vi "Convert Error Cluster to Table.vi"(11 "Error Codes":cluster{i32, string}[](array[cluster])) -> (2 "Code":i32[](array[numeric]), 3 "String":string[](array[string]))   [LabVIEW 2019, in "Protection and Counter Addon System Explorer.lvlib"] (continued)
 application instance."}, {1501, "LabVIEW: (Hex 0x5DD) Not a VRML 97 file, or contains unsupported models."}, {1502, "LabVIEW: (Hex 0x5DE) Cannot save a bad VI without its block diagram."}, {1503, "LabVIEW: (Hex 0x5DF) Cannot save a clone of a reentrant VI."}, {1504, "LabVIEW: (Hex 0x5E0) Cannot save a remote panel."}, {1505, "LabVIEW: (Hex 0x5E1) Cannot save a remote-debugging VI."}, {1506, "LabVIEW: (Hex 0x5E2) Cannot save a VI that is being edited in another context."}, {1507, "LabVIEW: (Hex 0x5E3) Cannot change the name or path of a VI in its current state."}, {1508, "LabVIEW: (Hex 0x5E4) Cannot change the name or path of a VI that is part of a library in its current state."}, {1509, "LabVIEW: (Hex 0x5E5) The response from the NI Service Locator is not a valid HTTP response."}, {1510, "LabVIEW: (Hex 0x5E6) The requested service was not found as a registered service with the NI Service Locator."}, {1511, "LabVIEW: (Hex 0x5E7) The requested service is a registered service with the NI Service Locator but it did not contain a port mapping."}, {1512, "LabVIEW: (Hex 0x5E8) trying to set indexes of bundle/unbundle with an array that is too long"}, {1513, "LabVIEW: (Hex 0x5E9) trying to set indexes of bundle/unbundle with an array that is too short"}, {1514, "LabVIEW: (Hex 0x5EA) trying to set index of bundle/unbundle to an element not in the cluster"}, {1515, "LabVIEW: (Hex 0x5EB) Cannot access this property because the conditional terminal has not been created."}, {1516, "LabVIEW: (Hex 0x5EC) The method in the DLL overwrote the space allocated for one of its parameters. This may have corrupted memory."}, {1517, "LabVIEW: (Hex 0x5ED) An error occurred in the Call Library Node processing. This error was most likely a configuration mismatch between the calling conventions of the Call Library Node and the function being called in the DLL."}, {1518, "LabVIEW: (Hex 0x5EE) Cannot find default printer. Make sure you have installed and selected a default printer."}, {1519, "LabVIEW: (Hex 0x5EF) Unable to print. Make sure you have installed a printer."}, {1520, "LabVIEW: (Hex 0x5F0) Font not found. LabVIEW cannot find the font at the specified path, or the font is not a True Type (.ttf) font."}, {1521, "LabVIEW: (Hex 0x5F1) Cannot read the value of a control that contains placeholder data."}, {1522, "LabVIEW: (Hex 0x5F2) You can write the Data Binding:Path property only if the control is already bound to a PSP URL."}, {1523, "LabVIEW: (Hex 0x5F3) Passed an invalid number of strings to the Strings [ ] property. You must pass either 1 string or 6 strings."}, {1524, "LabVIEW: (Hex 0x5F4) The target version for save is not formatted correctly."}, {1525, "LabVIEW: (Hex 0x5F5) You cannot read the value of a control when the class that defines the data is not available. You must load a missing LabVIEW class file to make this data readable."}, {1526, "LabVIEW: (Hex 0x5F6) This property does not apply when the plot legend of a graph or chart is in tree view."}, {1527, "LabVIEW: (Hex 0x5F7) Attempted to read flattened data of a LabVIEW class that is not currently loaded into LabVIEW."}, {1528, "LabVIEW: (Hex 0x5F8) A scene object with the specified name was not found."}, {1529, "LabVIEW: (Hex 0x5F9) There are too many nested VI calls. This typically results from recursion without a proper termination condition to stop the recursion."}, {1530, "LabVIEW: (Hex 0x5FA) The running VI attempted to make a subVI call into a top-level VI. LabVIEW does not allow calls into top-level VIs."}, {1531, "LabVIEW: (Hex 0x5FB) The LabVIEW class data cannot be unflattened because the class is broken. You must fix problems with the class before LabVIEW can unflatten data of this class."}, {1532, "LabVIEW: (Hex 0x5FC) The target application instance is currently being destroyed. You cannot get a new reference to the application instance or load a VI in the application instance."}, {1533, "LabVIEW: (Hex 0x5FD) A shared variable node cannot be created from the specified terminal."}, {1534, "LabVIEW: (Hex 0x5FE) The semaphore you specified does not exist. LabVIEW cannot return a reference to the semaphore."}, {1535, "LabVIEW: (Hex 0x5FF) The semaphore reference you specified is invalid."}, {1536, "LabVIEW: (Hex 0x600) To save a password-protected VI for a previous LabVIEW version, you must enter the password."}, {1537, "LabVIEW: (Hex 0x601) Member VI is not dynamic dispatch."}, {1538, "LabVIEW: (Hex 0x602) To perform this operation you must have the LabVIEW Statechart Module installed."}, {1539, "LabVIEW: (Hex 0x603) Valid stipple factors are 1 - 256"}, {1540, "LabVIEW: (Hex 0x604) Cannot pass a degenerate vector for the normal of an object."}, {1541, "LabVIEW: (Hex 0x605) This property or method is not valid because the object is not billboarded."}, {1542, "LabVIEW: (Hex 0x606) You must set the drawable of the object before you configure billboard parameters."}, {1543, "LabVIEW: (Hex 0x607) Cannot pass an empty position list for billboarding."}, {1544, "LabVIEW: (Hex 0x608) LabVIEW attempted a read, write, or seek on a file opened in unbuffered mode, and the data size is not a multiple of the disk sector size."}, {1545, "LabVIEW: (Hex 0x609) LabVIEW attempted to read or write data to a file opened in unbuffered mode, and the data is not aligned properly."}, {1546, "LabVIEW: (Hex 0x60A) The VI must be in a project to use this property."}, {1547, "LabVIEW: (Hex 0x60B) There was an error generating the type library."}, {1548, "LabVIEW: (Hex 0x60C) Queue refnum cannot be obtained with a size of zero. Size input must be a positive number or -1 for unlimited size."}, {1549, "LabVIEW: (Hex 0x60D) An unexpected error occurred during statechart code generation."}, {1550, "LabVIEW: (Hex 0x60E) The license for the I/O server type is invalid."}, {1553, "LabVIEW: (Hex 0x611) The LabVIEW Run-Time Engine cannot load the polymorphic VI. This error occurs in stand-alone applications when the VI is polymorphic."}, {1554, "LabVIEW: (Hex 0x612) The current LabVIEW target cannot load control VIs."}, {1555, "LabVIEW: (Hex 0x613) Property or invoke node is corrupt."}, {1556, "LabVIEW: (Hex 0x614) The reference is invalid. This error might occur because the reference has been deleted."}, {1557, "LabVIEW: (Hex 0x615) LabVIEW tried to access duplicate references at the same time."}, {1558, "LabVIEW: (Hex 0x616) There is a type mismatch between the wire type and the internal data type of the reference. This problem might occur due to a type cast error."}, {1559, "LabVIEW: (Hex 0x617) You cannot use Open VI Reference to create a reference to a VI that the creating VI accesses through community scope."}, {1560, "LabVIEW: (Hex 0x618) A library cannot list itself as a friend."}, {1561, "LabVIEW: (Hex 0x619) A library cannot list an item from a foreign application instance as a friend."}, {1562, "LabVIEW: (Hex 0x61A) The specified project or library is locked."}, {1563, "LabVIEW: (Hex 0x61B) LabVIEW did not generate documentation files for the statechart. Ensure all configuration windows are closed."}, {1564, "LabVIEW: (Hex 0x61C) Project file cannot be saved at this time. The project has a locked untitled dependency. The lock prevents giving the untitled item a name so it cannot be saved."}, {1565, "LabVIEW: (Hex 0x61D) LabVIEW cannot save the library file at this time. The library has a locked untitled dependency. The lock prevents giving the untitled item a name, which is required to save the library file."}, {1566, "LabVIEW: (Hex 0x61E) LabVIEW cannot save the untitled library file at this time. The library is locked. The lock prevents giving the untitled library a name, which is required to save the library."}, {1567, "LabVIEW: (Hex 0x61F) The control is not located in the same VI as the control reference."}, {1568, "LabVIEW: (Hex 0x620) This method requires Excel to be installed."}, {1569, "LabVIEW: (Hex 0x621) This method requires DIAdem 8.1 or later to be installed."}, {1570, "LabVIEW: (Hex 0x622) This method requires the array to be of numeric or string type."}, {1571, "LabVIEW: (Hex 0x623) You cannot open a packed library saved in a version earlier than the current version of LabVIEW."}, {1572, "LabVIEW: (Hex 0x624) The long name of the property is not unique."}, {1573, "LabVIEW: (Hex 0x625) You cannot load a packed library built for a target or operating system different than the current target or operating system."}, {1574, "LabVIEW: (Hex 0x626) Cannot open a file with separated compiled code in the LabVIEW Run-Time Engine."}, {1575, "LabVIEW: (Hex 0x627) The function name for the %s node cannot be found in the library. To correct this error, right-click the Call Library Function Node and select Configure from the shortcut menu. Then choose the correct function name."}, {1576, "LabVIEW: (Hex 0x628) A Start Asynchronous Call node received a reference input that was not configured to allow asynchronous calls. To fix this error, include either the 0x80 option flag or the 0x100 option flag when you open the reference with the Open VI Reference function."}, {1577, "LabVIEW: (Hex 0x629) A Wait On Asynchronous Call node received a reference input that was not configured to wait on an asynchronous call. To fix this error, include the 0x100 option flag when you open the VI reference with the Open VI Reference function."}, {1578, "LabVIEW: (Hex 0x62A) Asynchronous calls are not allowed on remote VI references."}, {1579, "LabVIEW: (Hex 0x62B) Specified paths do not share a common directory."}, {1580, "LabVIEW: (Hex 0x62C) Cannot find the compiled code in the compiled object cache."}, {1581, "LabVIEW: (Hex 0x62D) Cannot use this property on either .NET or ActiveX Container."}, {1582, "LabVIEW: (Hex 0x62E) Cannot call (Target)SaveInstrument on an Inline VI with Save Level greater than 0."}, {1583, "LabVIEW: (Hex 0x62F) LabVIEW Real-Time target is already connected to a host VI. You cannot initiate a remote panel connection to a Real-Time target while also using a host VI to connect to the target. Choose only one method to connect to the target."}, {1584, "LabVIEW: (Hex 0x630) The data in the reference cannot be resized. There is a size mismatch between the data in the reference and the data wired to the Data Value Reference Write Element border node."}, {1585, "LabVIEW: (Hex 0x631) The class library is loaded, but its datatype is not ready to be instantiated."}, {1586, "LabVIEW: (Hex 0x632) Compiled code is out of date."}, {1587, "LabVIEW: (Hex 0x633) VI is not marked to separate compiled code from source file."}, {1588, "LabVIEW: (Hex 0x634) Compiled object cache is corrupt."}, {1589, "LabVIEW: (Hex 0x635) The loaded .NET assembly was not found in its original directory."}, {1590, "LabVIEW: (Hex 0x636) The qualified name of one of the dependencies of the specified file is not what LabVIEW expected. This mismatch implies that the dependency report is unreliable, so the ReadLinkInfo operation was aborted."}, {1591, "LabVIEW: (Hex 0x637) The 0x40 option flag is not valid for either the target VI or the other option flags of the Open VI Reference function."}, {1592, "LabVIEW: (Hex 0x638) The asynchronous option flags require a strictly typed VI reference for the type specifier input of the Open VI Reference function."}, {1593, "LabVIEW: (Hex 0x639) Only one asynchronous call option can be passed into an Open VI Reference at a time."}, {1594, "LabVIEW: (Hex 0x63A) This VI type does not support inlining."}, {1595, "LabVIEW: (Hex 0x63B) The RT target does not have enough memory to load the startup application."}, {1596, "LabVIEW: (Hex 0x63C) Cannot use SSL on this operating system because SSL is either not configured, not installed, or not supported."}, {1597, "LabVIEW: (Hex 0x63D) The Paste Data operation attempted to paste data into a destination that would have had a dimmed 'paste' option in the shortcut menu."}, {1598, "LabVIEW: (Hex 0x63E) The requested path does not match a LabVIEW class in memory."}, {1599, "LabVIEW: (Hex 0x63F) An empty string is not a valid method name."}, {1600, "LabVIEW: (Hex 0x640) The specified method was not found on the specified LabVIEW class."}, {1601, "LabVIEW: (Hex 0x641) Although the requested class (or one of its ancestors) does have a member VI of the requested name, that VI is not actually a method. Either it has no input terminal of the class type or it is a non-runnable kind of VI, like a global VI, control VI, or poly VI."}, {1602, "LabVIEW: (Hex 0x642) The value supplied for the enum input is not supported on this method or property."}, {1603, "LabVIEW: (Hex 0x643) The Open VI Reference function does not support using an asynchronous call by reference option with the <b>Prepare for reentrant run</b> option."}, {1604, "LabVIEW: (Hex 0x644) The Open VI Reference function does not support using the option 0x08 (<b>Prepare for reentrant run</b>) with the asynchronous call by reference options 0x80 (<b>Prepare to call and forget</b>) or 0x100 (<b>Prepare to call and collect</b>)."}, {1605, "LabVIEW: (Hex 0x645) A process attempted to send a message with an invalid priority."}, {1606, "LabVIEW: (Hex 0x646) While attempting to launch, an actor's <b>Pre Launch Init</b> method failed."}, {1607, "LabVIEW: (Hex 0x647) Invalid message enqueuer wired to Actor.lvclass:Launch Actor.vi."}, {1608, "LabVIEW: (Hex 0x648) This actor stopped because it received an emergency stop message."}, {1609, "LabVIEW: (Hex 0x649) This class cannot load into this application instance."}, {1610, "LabVIEW: (Hex 0x64A) The To-Caller and To-Self queues for this actor already are initialized."}, {1611, "LabVIEW: (Hex 0x64B) An internal error occurred because a front panel item has no execute data. Recompiling the VI may fix this issue."}, {1612, "LabVIEW: (Hex 0x64C) You attempted to invoke a dynamic dispatch VI statically. The object you supplied for the dynamic dispatch terminal has an override VI for the chosen method that is not the same as the VI you specified. LabVIEW does not allow callers to directly invoke ancestor versions of the object's method."}, {1613, "LabVIEW: (Hex 0x64D) Calls to remote application instances are not supported for dynamic dispatch VIs."}, {1614, "LabVIEW: (Hex 0x64E) LabVIEW could not create a class with the name you specified. A class with that name already exists."}, {1615, "LabVIEW: (Hex 0x64F) LabVIEW cannot build a path to an .rtm file from the VI being saved."}, {1616, "LabVIEW: (Hex 0x650) The path to save the report is not valid. A valid path cannot contain any of the following characters: <b>(Windows)</b> < > / | : \" * ? or <b>(OS X/Linux)</b> < > \\ | : \" * ?."}, {1617, "LabVIEW: (Hex 0x651) LabVIEW is unable to generate a VI comparison report. Make sure you have write permission to the path you specified and generate the report again."}, {1619, "LabVIEW: (Hex 0x653) LabVIEW is unable to find the Microsoft Word components. Make sure you installed Microsoft Word correctly."}, {1620, "LabVIEW: (Hex 0x654) LabVIEW is unable to create the Microsoft Word report. Try generating the report again. If the problem persists, contact National Instruments technical support."}, {1621, "LabVIEW: (Hex 0x655) LabVIEW is unable to create the Microsoft Word report. Try generating the report again. If the problem persists, contact National Instruments technical support."}, {1622, "LabVIEW: (Hex 0x656) LabVIEW is unable to create the Microsoft Word report. Make sure you installed Microsoft Word correctly and create the report again."}, {1623, "LabVIEW: (Hex 0x657) LabVIEW is unable to find the Microsoft Word components. Make sure you installed Microsoft Word correctly."}, {1624, "LabVIEW: (Hex 0x658) You can only generate web page or plain text reports on OS X and Linux."}, {1625, "LabVIEW: (Hex 0x659) LabVIEW is unable to create a report in the format that you specify. Make sure the report file extension that you entered is one of the following extensions: .xml, .txt, and <b>(Windows)</b> .doc."}, {1626, "LabVIEW: (Hex 0x65A) Unable to disconnect this control from the type definition. The type definition may belong to a library that requires activation."}, {1627, "LabVIEW: (Hex 0x65B) The control index at position %d is invalid."}, {1628, "LabVIEW: (Hex 0x65C) LabVIEW cannot convert the input data type at position %d to the control data type."}, {1629, "LabVIEW: (Hex 0x65D) The control must have a terminal on the block diagram.."}, {1630, "LabVIEW: (Hex 0x65E) If you wire a variant or a LabVIEW class library file (.lvclass) to this function, you must call the function on a VI in the same application instance."}, {1631, "LabVIEW: (Hex 0x65F) Library not found. This VI does not belong to a library, or the library was removed from disk."}, {1632, "LabVIEW: (Hex 0x660) You cannot insert a custom control directly into a subpanel. Use a VI with the custom control on its front panel instead."}, {1633, "LabVIEW: (Hex 0x661) The LabVIEW Real-Time process encountered an unexpected error and restarted automatically."}, {1634, "LabVIEW: (Hex 0x662) The debug feature of the Actor Framework to automatically open the front panel of the Actor Core VI is not supported in the run-time engine. You must add code to your actor's Actor Core VI to open and close its own panel."}, {1635, "LabVIEW: (Hex 0x663) LabVIEW failed to invoke the Xcode toolchain. Make sure you installed Xcode properly and have signed the Xcode license agreement."}, {1636, "LabVIEW: (Hex 0x664) The SSE settings of the target or operating system does not match the settings of a VI in the application you are trying to build. That VI cannot recompile because it does not have a block diagram."}, {1637, "LabVIEW: (Hex 0x665) This operation cannot be performed on reentrant clone VIs."}, {1638, "LabVIEW: (Hex 0x666) Muliple errors occurred upstream. No details are available (error information may have been deleted somewhere along the way)."}, {1639, "LabVIEW: (Hex 0x667) The test harness actor executed for longer time than the timeout specified. It was stopped with an Emergency Stop message."}, {1640, "LabVIEW: (Hex 0x668) Channels are incompatible with asynchronous call by reference options 0x80 (<b>Prepare for call-and-forget</b>) and 0x100 (<b>Prepare for call-and-collect</b>)."}, {1641, "LabVIEW: (Hex 0x669) LabVIEW was asked to create a channel for an undefined type, such as an array with no subtype or a missing typedef."}, {1642, "LabVIEW: (Hex 0x66A) LabVIEW attempted to recreate a missing channel endpoint, but the channel template does not have an endpoint of this name. The channel template may have been edited to remove support for this endpoint."}, {1643, "LabVIEW: (Hex 0x66B) The requested channel template does not support the requested transmission type. Some channels only support types that have specific abilities. For example, the Accumulator requires a numeric type so the values may be added up. This error also may occur if the channel template itself is flawed and producing broken code for all requested types."}, {1644, "LabVIEW: (Hex 0x66C) The new name used to rename is the same as the name of data already existing in group."}, {1645, "LabVIEW: (Hex 0x66D) The input data does not exist."}, {1646, "LabVIEW: (Hex 0x66E) The source element type cannot be converted to the destination element type."}, {1647, "LabVIEW: (Hex 0x66F) The plot type cannot be mapped to TDMS channels."}, {1648, "LabVIEW: (Hex 0x670) This VI halted execution when attempting to read from or write to a channel wire. The channel includes a branch not connected to a channel endpoint. All branches of a channel wire must be connected to a channel endpoint, either in this block diagram or in the block diagram of a calling VI if the channel is passed out through the connector pane."}, {1649, "LabVIEW: (Hex 0x671) The data carried by a channel wire must be of a public data type. You are trying to create a channel of a typedef or class that uses an access scope other than public or is inside a non-public library."}, {1650, "LabVIEW: (Hex 0x672) LabVIEW.exe not found. Make sure the configured LabVIEW is present under Program Files/Program Files(x86)->National Instruments-><Specific LabVIEW version>->LabVIEW.exe."}, {1651, "LabVIEW: (Hex 0x673) Other instances of LabVIEW might be open and holding the network resources. Close all instances of the configured LabVIEW and try again."}, {1652, "LabVIEW: (Hex 0x674) The network connection was closed. This can happen if the LabVIEW process is killed manually or the firewall restricted/closed the network connection."}, {1653, "LabVIEW: (Hex 0x675) The configured VI is not found. Reconfigure the VI Interop node to point to proper location."}, {1654, "LabVIEW: (Hex 0x676) Failed to launch LabVIEW. Make sure you can run configured LabVIEW. Contact National Instruments for technical support."}, {1655, "LabVIEW: (Hex 0x677) VI Interop node did not execute as expected. Contact National Instruments for technical support."}, {1656, "LabVIEW: (Hex 0x678) Connector pane of the configured VI has changed since VI Interop node was configured. Try reloading the caller VI."}, {1657, "LabVIEW: (Hex 0x679) The component reference is invalid."}, {1658, "LabVIEW: (Hex 0x67A) A Type Specialization structure cannot be assigned a default frame. The last frame will be used if all earlier frames are broken."}, {1659, "LabVIEW: (Hex 0x67B) A Type Specialization structure cannot have conditions assigned to its frames."}, {1660, "LabVIEW: (Hex 0x67C) Cannot set the Active Frame property on a Type Specialization structure. The Active Frame is computed automatically by choosing the first unbroken frame, defaulting to the last frame if all are broken."}, {1661, "LabVIEW: (Hex 0x67D) The NI Python Interface DLL niPythonInterface.dll could not be loaded."}, {1662, "LabVIEW: (Hex 0x67E) The NI Python Host EXE niPythonHost.exe could not be found."}, {1663, "LabVIEW: (Hex 0x67F) Unable to load the Python interpreter of the specified version. Ensure that you install the supported versions of Python, and the bitness of Python matches the bitness of LabVIEW that opens the Python session."}, {1664, "LabVIEW: (Hex 0x680) The specified Python version is not supported."}, {1665, "LabVIEW: (Hex 0x681) The specified Python path is not valid."}, {1666, "LabVIEW: (Hex 0x682) The Python session refnum input is not valid."}, {1667, "LabVIEW: (Hex 0x683) The specified Python module could not be imported."}, {1668, "LabVIEW: (Hex 0x684) The specified Python function could not be found in the specified module."}, {1669, "LabVIEW: (Hex 0x685) The operation to convert from LabVIEW objects to Python objects failed."}, {1670, "LabVIEW: (Hex 0x686) The operation to convert from Python objects to LabVIEW objects failed."}, {1671, "LabVIEW: (Hex 0x687) There was an error in executing the specified function."}, {1672, "LabVIEW: (Hex 0x688) There was an unknown Python error in the operation."}, {1673, "LabVIEW: (Hex 0x689) The VI is not loaded in memory. To load the VI into memory on the server, manually open the VI or use Open VI Reference."}, {1674, "LabVIEW: (Hex 0x68A) The peer closed the network connection. To configure access on the server side for the machine, navigate to Tools>>Options>>VI Server."}, {1675, "LabVIEW: (Hex 0x68B) The input string contains one or more invalid UTF-8 string sequences."}, {1676, "LabVIEW: (Hex 0x68C) A Start Asynchronous Call node received a reference input that is not configured to allow asynchronous calls. When you open the reference with the Open VI Reference node, select \"Prepare for asynchronous call without wait\" or \"Prepare for asynchronous call with wait\"."}, {1677, "LabVIEW: (Hex 0x68D) A Wait On Asynchronous Call node received a reference input that is not configured to wait on an asynchronous call. When you open the VI reference with the Open VI Reference node, select \"Prepare for asynchronous call with wait\"."}, {1678, "LabVIEW: (Hex 0x68E) EnableSimultaneousCalls is not valid for either the target VI or the other call options of the Open VI Reference."}, {1679, "LabVIEW: (Hex 0x68F) Component of the specified name is not in memory."}, {1680, "LabVIEW: (Hex 0x690) The text read from the file contains one or more invalid UTF-8 string sequences."}, {1681, "LabVIEW: (Hex 0x691) Operation attempted to update element, key, or value data in set or map controls. No data operation is allowed for controls inside a set or map."}, {1682, "LabVIEW: (Hex 0x692) The string contains an unexpected null character."}, {1690, "LabVIEW: (Hex 0x69A) Cannot insert the panel of a VI in a panel container if the VI is not running."}, {1691, "LabVIEW: (Hex 0x69B) Cannot insert the panel of a VI in a panel container if the panel is already displayed in a window or another panel container."}, {1692, "LabVIEW: (Hex 0x69C) Inserting this panel results in a cyclic dependency between panel containers."}, {1800, "LabVIEW: (Hex 0x708) Start time input is not an integer multiple of dt. Value was coerced to nearest integer multiple of dt."}, {1801, "LabVIEW: (Hex 0x709) Duration input is not an integer multiple of dt. Value was coerced to nearest integer multiple of dt."}, {1802, "LabVIEW: (Hex 0x70A) Waveforms have different dt values."}, {1803, "LabVIEW: (Hex 0x70B) Waveform x-axis value requested is out of range."}, {1804, "LabVIEW: (Hex 0x70C) Start index, value, or tolerance is NaN."}, {1805, "LabVIEW: (Hex 0x70D) Start index is out of range."}, {1806, "LabVIEW: (Hex 0x70E) Signal value input is outside the range of the digital data."}, {1807, "LabVIEW: (Hex 0x70F) Appending data with mismatched numbers of digital samples or signals."}, {1808, "LabVIEW: (Hex 0x710) Values other than 0, 1, L, H are present in the digital data."}, {1809, "LabVIEW: (Hex 0x711) Highest resolution supported for conversion is 52."}, {1814, "LabVIEW: (Hex 0x716) Values other than 0, 1, L, and H are present in the digital data and were coerced to 0."}, {2300, "LabVIEW: (Hex 0x8FC) The model code of the target is different than the model code of the image."}, {2301, "LabVIEW: (Hex 0x8FD) The image is invalid."}, {2302, "LabVIEW: (Hex 0x8FE) The operation cannot be completed because the target is locked."}, {2303, "LabVIEW: (Hex 0x8FF) The version of the image is not compatible with the version of the system replication VIs."}, {2304, "LabVIEW: (Hex 0x900) The command is not supported on the target."}, {2305, "LabVIEW: (Hex 0x901) The target did not restart because it is already in Install Mode."}, {2306, "LabVIEW: (Hex 0x902) The format command failed. If your target has a Safe Mode dip switch, make sure that it is enabled and try the format command again."}, {2307, "LabVIEW: (Hex 0x903) Failed to remove files or folders."}, {2308, "LabVIEW: (Hex 0x904) Found no configured network adapters."}, {2535, "LabVIEW: (Hex 0x9E7) Data from TDMS files is read using the byte order of the host system. Byte order settings that differ from the host order are ignored."}, {2552, "LabVIEW: (Hex 0x9F8) This property does not contain data."}, {2901, "LabVIEW: (Hex 0xB55) The source control operation was cancelled before completion."}, {2902, "LabVIEW: (Hex 0xB56) A change occurred to the specified file while the operation was running. Reload the file."}, {4800, "LabVIEW: (Hex 0x12C0) Selected Device is Invalid"}, {4801, "LabVIEW: (Hex 0x12C1) Invalid sound task refnum."}, {4802, "LabVIEW: (Hex 0x12C2) The sound device is busy."}, {4803, "LabVIEW: (Hex 0x12C3) The sound driver or card cannot accommodate the specified configuration.  Check that the parameters entered are within the supported range for the hardware and drivers."}, {4804, "LabVIEW: (Hex 0x12C4) Cannot write in file playback."}, {4805, "LabVIEW: (Hex 0x12C5) Could not find the sound file."}, {4806, "LabVIEW: (Hex 0x12C6) DirectX 8.0 or higher is required to run."}, {4810, "LabVIEW: (Hex 0x12CA) Cannot recognize sound format."}, {4811, "LabVIEW: (Hex 0x12CB) Cannot support sound format."}, {4820, "LabVIEW: (Hex 0x12D4) A buffer underflow has occurred."}, {4821, "LabVIEW: (Hex 0x12D5) Overwrite error."}, {4822, "LabVIEW: (Hex 0x12D6) A timeout occurred before the operation finished."}, {4823, "LabVIEW: (Hex 0x12D7) You cannot perform this operation without an active task.  Ensure that a task is active and try again. An input task might stop running if the input buffer overflows. Overflow occurs when the data is not read fast enough."}, {14001, "LabVIEW: (Hex 0x36B1) Invalid refnum."}, {14002, "LabVIEW: (Hex 0x36B2) Invalid string."}, {14003, "LabVIEW: (Hex 0x36B3) A request for a synchronous advise transaction has timed out."}, {14004, "LabVIEW: (Hex 0x36B4) The response to the transaction caused the DDE_FBUSY bit to be set."}, {14005, "LabVIEW: (Hex 0x36B5) A request for a synchronous data transaction has timed out."}, {14006, "LabVIEW: (Hex 0x36B6) The DDEML function was called without first calling the DdeInitialize function or an invalid instance identifier was pass to a DDEML function."}, {14007, "LabVIEW: (Hex 0x36B7) An application initialized as APPCLASS_MONITOR has attempted to perform a DDE transaction, or an application initialized as APPCMD_CLIENTONLY has attempted to perform server transactions."}, {14008, "LabVIEW: (Hex 0x36B8) A request for a synchronous execute transaction has timed out."}, {14009, "LabVIEW: (Hex 0x36B9) A parameter failed to be validated by the DDEML:  e.g., the data handle is initialized with a different name-item  or different clipboard data format than that required; the application used a client-side conversation handle with a server-side function, or vice-versa; the application used a freed data or string handle; or more than one instance of the application used the same object."}, {14010, "LabVIEW: (Hex 0x36BA) A DDEML application has created a prolonged race condition (where the server application outruns the client), causing large amounts of memory to be consumed."}, {14011, "LabVIEW: (Hex 0x36BB) A memory allocation failed."}, {14012, "LabVIEW: (Hex 0x36BC) A transaction failed."}, {14013, "LabVIEW: (Hex 0x36BD) A client's attempt to establish a conversation has failed."}, {14014, "LabVIEW: (Hex 0x36BE) A request for a synchronous poke transaction has timed out."}, {14015, "LabVIEW: (Hex 0x36BF) An internal call to the PostMessage function has failed."}, {14016, "LabVIEW: (Hex 0x36C0) An application instance with a synchronous transaction already in progress attempted to initiate another synchronous transaction, or the DdeEnableCallback function was called from within a DDEML call function."}, {14017, "LabVIEW: (Hex 0x36C1) A server-side transaction was attempted on a conversation that was terminated by the client, or the server terminated before completing a transaction."}, {14018, "LabVIEW: (Hex 0x36C2) An internal error has occurred in the DDEML."}, {14019, "LabVIEW: (Hex 0x36C3) A request to end an advise transaction has timed out."}, {14020, "LabVIEW: (Hex 0x36C4) An invalid transaction identifier was passed to a DDEML function.  After the application has returned from an XTYP_XACT_COMPLETE callback, the transaction identifier for that callback is no longer valid."}, {14021, "LabVIEW: (Hex 0x36C5) Invalid command code."}, {14022, "LabVIEW: (Hex 0x36C6) Occurrence timeout; the transaction timed out before it completed."}, {14050, "LabVIEW: (Hex 0x36E2) ActiveX Event data was not available."}, {14051, "LabVIEW: (Hex 0x36E3) ActiveX Event Information was not available."}, {14052, "LabVIEW: (Hex 0x36E4) The occurrence associated with the ActiveX Event was not found."}, {14053, "LabVIEW: (Hex 0x36E5) The ActiveX Event queue could not be created."}, {16211, "LabVIEW: (Hex 0x3F53) 211 System status or system help reply."}, {16214, "LabVIEW: (Hex 0x3F56) 214 Help message."}, {16220, "LabVIEW: (Hex 0x3F5C) 220 \"domain\" Service ready."}, {16221, "LabVIEW: (Hex 0x3F5D) 221 domain service closing transmission channel."}, {16250, "LabVIEW: (Hex 0x3F7A) 250 Requested mail action okay, completed."}, {16251, "LabVIEW: (Hex 0x3F7B) 251 User not local; will forward to \"forward-path.\""}, {16354, "LabVIEW: (Hex 0x3FE2) 354 Start mail input; end with two carriage-return/line-feed characters."}, {16421, "LabVIEW: (Hex 0x4025) 421 \"domain\" service not available, closing transmission channel. This might be a reply to any command if the service knows it must shut down."}, {16450, "LabVIEW: (Hex 0x4042) 450 Requested mail action not taken: mailbox unavailable. For example, the mailbox might be busy."}, {16451, "LabVIEW: (Hex 0x4043) 451 Requested action aborted: local error in processing."}, {16452, "LabVIEW: (Hex 0x4044) 452 Requested action not taken: insufficient system storage."}, {16500, "LabVIEW: (Hex 0x4074) 500 Syntax error, command unrecognized. For example, the command line might be too long."}, {16501, "LabVIEW: (Hex 0x4075) 501 Syntax error in parameters or arguments."}, {16502, "LabVIEW: (Hex 0x4076) 502 Command not implemented."}, {16503, "LabVIEW: (Hex 0x4077) 503 Bad sequence of commands."}, {16504, "LabVIEW: (Hex 0x4078) 504 Command parameter not implemented."}, {16550, "LabVIEW: (Hex 0x40A6) 550 Requested action not taken: mailbox unavailable. For example, the mailbox was not found or there is no access."}, {16551, "LabVIEW: (Hex 0x40A7) 551 User not local; try \"forward-path.\""}, {16552, "LabVIEW: (Hex 0x40A8) 552 Requested mail action aborted: exceeded storage allocation."}, {16553, "LabVIEW: (Hex 0x40A9) 553 Requested action not taken: mailbox name not allowed. For example, the mailbox syntax might be incorrect."}, {16554, "LabVIEW: (Hex 0x40AA) 554 Transaction failed."}, {20338, "LabVIEW: (Hex 0x4F72) The number of signals in Input Signal A does not match the number of signals in Input Signal B. Unmatched signals will be ignored."}, {40620, "LabVIEW: (Hex 0x9EAC) One of the following conditions occurred: 1) This slot-based variable has already been read within this network cycle. 2) This shared-memory-based variable has never been instantiated by the owner."}, {40621, "LabVIEW: (Hex 0x9EAD) The source node is still online, but no new data has been received for more than one network cycle because no new data has been written to the channel on the source node."}, {40622, "LabVIEW: (Hex 0x9EAE) No new data has been received for more than one network cycle because the source node is offline."}, {40623, "LabVIEW: (Hex 0x9EAF) One of the values received from the source node was not read and was overwritten."}, {40624, "LabVIEW: (Hex 0x9EB0) One of the values was overwritten before it was sent.  LabVIEW returns this warning for non-shared memory variables that have been written more than once in a single network cycle."}, {40625, "LabVIEW: (Hex 0x9EB1) No data was sent from this channel in the previous network cycle because a write operation was delayed beyond a preconfigured threshold.  An interrupt probably caused the delay."}, {40626, "LabVIEW: (Hex 0x9EB2) Clock synchronization algorithm failed because a sufficient number of cycle-start packets were missed. No additional write network transactions are allowed until the deterministic-communication engine is restarted."}, {40628, "LabVIEW: (Hex 0x9EB4) Attempted read operation at least twice before it succeeded due to new data being placed into the buffer."}, {40630, "LabVIEW: (Hex 0x9EB6) Network transmission violated requested timing.  Refer to the \"Avoid Jitter\" topic and other timing topics in the LabVIEW Help for more information about what might have caused this error and how to avoid it."}, {40631, "LabVIEW: (Hex 0x9EB7) A deployed configuration for one or more network nodes does not match the configuration for this node."}, {40632, "LabVIEW: (Hex 0x9EB8) Detected a valid packet on the network that does not conform to the National Instruments deterministic protocol.  The node or network will be shut down."}, {56000, "LabVIEW: (Hex 0xDAC0) Generic project error."}, {56001, "LabVIEW: (Hex 0xDAC1) An item with this name already exists in the project."}, {56002, "LabVIEW: (Hex 0xDAC2) An item with this path already exists in the project."}, {56003, "LabVIEW: (Hex 0xDAC3) Adding this item would cause a conflict with another item."}, {56004, "LabVIEW: (Hex 0xDAC4) The project item could not be found."}, {56005, "LabVIEW: (Hex 0xDAC5) The item type is not compatible with the target type."}, {56006, "LabVIEW: (Hex 0xDAC6) You cannot add a packed library to a project library."}, {56007, "LabVIEW: (Hex 0xDAC7) You cannot add to a LabVIEW class any item that is or is a member of a library, XControl, state chart, or other LabVIEW class."}, {66014, "LabVIEW: (Hex 0x101DE) The I/O variable accessor requested a timestamp, but this I/O device or channel is not configured for timestamps."}, {66030, "LabVIEW: (Hex 0x101EE) This I/O variable is referencing an I/O device or channel that is not active in the current I/O mode.  Data read may be stale or invalid and data written may not be sent to the output."}, {66410, "LabVIEW: (Hex 0x1036A) The variable's value is being forced."}, {66411, "LabVIEW: (Hex 0x1036B) The I/O variable is referencing I/O that has been taken offline by the user.  The value used may not be current."}, {66430, "LabVIEW: (Hex 0x1037E) The fault was cleared and the controller is no longer in Fault mode, but the controller was unable to re-enter Active mode and is now in Configuration mode."}, {66463, "LabVIEW: (Hex 0x1039F) The NI Scan Engine is running but there are no I/O drivers that use the scan engine."}, {66464, "LabVIEW: (Hex 0x103A0) The global time on the controller was altered, which might affect the period of an iteration of the NI Scan Engine."}, {67200, "LabVIEW: (Hex 0x10680) LabVIEW Web Services: Cannot modify http header or response after written to socket."}, {67201, "LabVIEW: (Hex 0x10681) LabVIEW Web Services: Required input string is empty."}, {67202, "LabVIEW: (Hex 0x10682) LabVIEW Web Services: No POST data available for input Request ID."}, {311100, "LabVIEW: (Hex 0x4BF3C) Unable to get the host name from the variable path. The IP address is used to generate the default process variable (PV) name."}, {311101, "LabVIEW: (Hex 0x4BF3D) The EPICS Server I/O server cannot support the specified data type. LabVIEW created a string type process variable."}, {311102, "LabVIEW: (Hex 0x4BF3E) The EPICS Server I/O server cannot support the data type of the shared variable. LabVIEW created a string type process variable."}, {311103, "LabVIEW: (Hex 0x4BF3F) Unable to get the data type of the shared variable. LabVIEW created a string type process variable."}, {314000, "LabVIEW: (Hex 0x4CA90) Not enough elements to read."}, {314001, "LabVIEW: (Hex 0x4CA91) Not enough free space to write."}, {314010, "LabVIEW: (Hex 0x4CA9A) The writer endpoint was destroyed before it received an acknowledgement from the reader endpoint that all data was received. The reader endpoint might not have received some data."}, {314050, "LabVIEW: (Hex 0x4CAC2) You specified the URL of a remote endpoint that does not exist."}, {314051, "LabVIEW: (Hex 0x4CAC3) The remote endpoint did not prompt a connection with the local endpoint. Make sure you specify the correct URL with the URL terminal of the remote endpoint."}, {314205, "LabVIEW: (Hex 0x4CB5D) The local endpoint did not receive a response from the remote endpoint before the timeout expired."}, {314210, "LabVIEW: (Hex 0x4CB62) The endpoint timed out before another endpoint prompted a connection with it."}, {363500, "LabVIEW: (Hex 0x58BEC) Failed to connect to the specified hostname.  Be sure the specified hostname is correct, the server is running and configured to accept remote requests."}, {363501, "LabVIEW: (Hex 0x58BED) Cannot access or open the specified filename.  Be sure the path is correct, the file exists, and that it is not locked by another user."}, {363502, "LabVIEW: (Hex 0x58BEE) The specified file name is invalid or does not exist."}, {363503, "LabVIEW: (Hex 0x58BEF) The HTTP client-side libraries (or one of its dependencies) failed to load."}, {363504, "LabVIEW: (Hex 0x58BF0) Invalid username or password combination."}, {363505, "LabVIEW: (Hex 0x58BF1) An error occured while converting a file stream to a fixed buffer."}, {363506, "LabVIEW: (Hex 0x58BF2) The certificate path or CA information of the local host is invalid."}, {363507, "LabVIEW: (Hex 0x58BF3) LabVIEW could not verify the authenticity of the server."}, {363508, "LabVIEW: (Hex 0x58BF4) The request was aborted by the caller."}, {363509, "LabVIEW: (Hex 0x58BF5) LabVIEW could not read the specified filename."}, {363510, "LabVIEW: (Hex 0x58BF6) An error occurred while writing to the socket."}, {363511, "LabVIEW: (Hex 0x58BF7) An error occurred while reading from the socket."}, {363512, "LabVIEW: (Hex 0x58BF8) An error occurred while uploading a file."}, {363513, "LabVIEW: (Hex 0x58BF9) An error occurred while sending data on the network."}, {363514, "LabVIEW: (Hex 0x58BFA) An error occurred while receiving data from the network."}, {363515, "LabVIEW: (Hex 0x58BFB) The file exceeds the size limit on the server."}, {363516, "LabVIEW: (Hex 0x58BFC) Client does not have access to the specified resource (access is forbidden)."}, {363517, "LabVIEW: (Hex 0x58BFD) Cannot find the remote file."}, {363518, "LabVIEW: (Hex 0x58BFE) The remote file already exists."}, {363519, "LabVIEW: (Hex 0x58BFF) Storage space limits on the server exceeded."}, {363520, "LabVIEW: (Hex 0x58C00) The server does not recognize the transfer encoding."}, {363521, "LabVIEW: (Hex 0x58C01) Number of redirects to other resources exceeded."}, {363522, "LabVIEW: (Hex 0x58C02) The network communication socket is not ready."}, {363523, "LabVIEW: (Hex 0x58C03) An unknown error occurred in the curl libraries."}, {363524, "LabVIEW: (Hex 0x58C04) The specified protocol is invalid or unsupported."}, {363525, "LabVIEW: (Hex 0x58C05) Failed to negotiate an encryption key from the server."}, {363526, "LabVIEW: (Hex 0x58C06) An error occurred when trying to encrypt the user data."}, {363527, "LabVIEW: (Hex 0x58C07) An error occurred when trying to decrypt the user data."}, {363528, "LabVIEW: (Hex 0x58C08) The specified request header does not exist."}, {363529, "LabVIEW: (Hex 0x58C09) The server closed the connection prematurely."}, {363530, "LabVIEW: (Hex 0x58C0A) Redirection to another URL was forbidden."}, {363531, "LabVIEW: (Hex 0x58C0B) Minimum must be less than maximum."}, {363532, "LabVIEW: (Hex 0x58C0C) The ActivePlot value is not valid."}, {363533, "LabVIEW: (Hex 0x58C0D) No Plot exists for the current ActivePlot value."}, {363534, "LabVIEW: (Hex 0x58C0E) The ActiveXScale value is not valid."}, {363535, "LabVIEW: (Hex 0x58C0F) No XScale exists for the current ActiveXScale value."}, {363536, "LabVIEW: (Hex 0x58C10) The ActiveYScale value is not valid."}, {363537, "LabVIEW: (Hex 0x58C11) No YScale exists for the current ActiveYScale value."}, {363538, "LabVIEW: (Hex 0x58C12) The ActiveCursor value is not valid."}, {363539, "LabVIEW: (Hex 0x58C13) No Cursor exists for the current ActiveCursor value."}, {363540, "LabVIEW: (Hex 0x58C14) Charts do not support the Value property at this time."}, {363541, "LabVIEW: (Hex 0x58C15) Charts do not support the ValueSignaling property at this time."}, {363542, "LabVIEW: (Hex 0x58C16) Name and Value must not be empty."}, {363543, "LabVIEW: (Hex 0x58C17) Values must be unique."}, {363544, "LabVIEW: (Hex 0x58C18) Display values must be unique."}, {363545, "LabVIEW: (Hex 0x58C19) The ActiveBus value is not valid."}, {363546, "LabVIEW: (Hex 0x58C1A) No Bus exists for the current ActiveBus value."}, {363547, "LabVIEW: (Hex 0x58C1B) Cannot set Size of this control."}, {363548, "LabVIEW: (Hex 0x58C1C) Cannot set Size of this control."}, {363549, "LabVIEW: (Hex 0x58C1D) The main control and its additional parts don't have common visual ancestor."}, {363550, "LabVIEW: (Hex 0x58C1E) Unable to get window size before window is open if size has not been set."}, {363551, "LabVIEW: (Hex 0x58C1F) XAxisIndex is out of bounds."}, {363552, "LabVIEW: (Hex 0x58C20) YAxisIndex is out of bounds."}, {363553, "LabVIEW: (Hex 0x58C21) Growonly is not supported by polar graph."}, {363554, "LabVIEW: (Hex 0x58C22) Display values must not be empty."}, {363555, "LabVIEW: (Hex 0x58C23) The ActiveTab value is not valid."}, {363556, "LabVIEW: (Hex 0x58C24) No Tab exists for the current ActiveTab value."}, {363557, "LabVIEW: (Hex 0x58C25) Unable to set the visible cell at the specified location."}, {363558, "LabVIEW: (Hex 0x58C26) Unable to set the position of a locked label."}, {363559, "LabVIEW: (Hex 0x58C27) Unable to set the size of a locked label."}, {363560, "LabVIEW: (Hex 0x58C28) Invalid reference."}, {363561, "LabVIEW: (Hex 0x58C29) Control must be dynamically added to delete."}, {363562, "LabVIEW: (Hex 0x58C2A) The property cannot be set. This object is read-only."}, {363563, "LabVIEW: (Hex 0x58C2B) If the cursor is watching multiple plots, the YPosition property cannot be set."}, {363650, "LabVIEW: (Hex 0x58C82) A network error has occurred. Possible reasons for this error include Cross-Origin Resource Sharing (CORS) configuration issues between the client and the target server or that the client cannot reach the target server. Due to browser security restrictions, detailed information about the cause of the network error cannot be provided. You may find specific details about the cause of the network error in the browser development tools console or in the LabVIEW output window."}, {363651, "LabVIEW: (Hex 0x58C83) Setting a header or header value resulted in an error, possibly due to an invalid character in a header or header value. Verify that each header and header value contains only valid characters."}, {363652, "LabVIEW: (Hex 0x58C84) This target does not support modification of the cookie file input. The browser manages saving cookies from an HTTP response and including cookies in HTTP requests on behalf of the user. The HTTP Client VIs cannot manipulate cookies directly. Set the cookie file input as either Not a path or an empty path for this target."}, {363653, "LabVIEW: (Hex 0x58C85) This target does not support modification of the verify server input. The browser manages settings related to validation of a server's identity and establishing secure connections. Set the verify server input to True for this target."}, {363654, "LabVIEW: (Hex 0x58C86) This target does not support usage of an output file. Set output file as either Not a path or an empty path for this target."}, {363655, "LabVIEW: (Hex 0x58C87) This target is not subject to Cross-Origin Resource Sharing (CORS) restrictions and cannot perform CORS configuration. Do not attempt to perform CORS configuration on this target."}, {363656, "LabVIEW: (Hex 0x58C88) This target does not support proxy server configuration using the HTTP Client VIs. The host browser or environment must be configured directly to change proxy server settings. Do not attempt to perform proxy server configuration on this target."}, {363657, "LabVIEW: (Hex 0x58C89) This target does not support SSL configuration using the HTTP Client VIs. The host browser or environment must be configured directly to change SSL settings. Do not attempt to perform SSL configuration on this target."}, {363700, "LabVIEW: (Hex 0x58CB4) An internal error occurred when setting a CURL option."}, {363701, "LabVIEW: (Hex 0x58CB5) An internal error occurred when setting a CURL form option."}, {363702, "LabVIEW: (Hex 0x58CB6) An internal error occurred when getting a CURL form option."}, {363703, "LabVIEW: (Hex 0x58CB7) An internal error occured. The authenticator object was unexpectedly null."}, {363798, "LabVIEW: (Hex 0x58D16) The HTTP client produced an unknown error."}, {374101, "LabVIEW: (Hex 0x5B555) Invalid value index for appending data."}, {389298, "LabVIEW: (Hex 0x5F0B2) The operation you want to perform is not implemented. Possible reasons: the descendant class does not implement one of the required member VIs in the ancestor Modbus class; the descendant class data is lost and LabVIEW executes a member VI in the ancestor Modbus class that does not provide an implementation. Contact National Instruments for technical support."}, {389299, "LabVIEW: (Hex 0x5F0B3) You configured this serial request as a broadcast. The Modbus slave does not respond to broadcasts. Contact National Instruments for technical support."}, {678010, "LabVIEW: (Hex 0xA587A) The given new actor cannot substitute for the current actor. The Substitute Actor method does not know how to make this substitution."}, {180093009, "LabVIEW: (Hex 0xABC0051) Item not found, but subscription succeeded."}, {1073479937, "LabVIEW: (Hex 0x3FFC0101) ID Query not supported."}, {1073479938, "LabVIEW: (Hex 0x3FFC0102) Reset not supported."}, {1073479939, "LabVIEW: (Hex 0x3FFC0103) Self-test not supported."}, {1073479940, "LabVIEW: (Hex 0x3FFC0104) Error Query not supported."}, {1073479941, "LabVIEW: (Hex 0x3FFC0105) Revision Query not supported"}, {-61512, "LabVIEW FPGA: The destination directory path cannot contain parentheses."}, {-61511, "LabVIEW FPGA: Unsupported file type."}, {-61510, "LabVIEW FPGA: Cannot access distributed RAM from different clock domains."}, {-61509, "LabVIEW FPGA: Unsupported number of elements per read or write on the current target."}, {-61508, "LabVIEW FPGA: Node not supported in single-cycle Timed Loops."}, {-61507, "LabVIEW FPGA: Peer-to-peer FIFOs are unsupported on the current target."}, {-61506, "LabVIEW FPGA: The FPGA VI configured for running in simulation mode contains controls or indicators with duplicate names. The Read/Write function cannot read from or write to controls or indicators with duplicate names. Rename the controls or indicators."}, {-61505, "LabVIEW FPGA: Unsupported .xci file."}, {-61504, "LabVIEW FPGA: Unsupported FIFO method."}, {-61503, "LabVIEW FPGA: Missing required Xilinx compilation tools."}, {-61502, "LabVIEW FPGA: File format mismatch."}, {-61501, "LabVIEW FPGA: Internal software error(s)."}, {-61500, "LabVIEW FPGA: An internal software error has occurred.  Please contact National Instruments technical support at ni.com/support with the following information:\n\nLabVIEW could not read a CLIP XML file."}, {-61499, "LabVIEW FPGA: An internal software error in the LabVIEW FPGA Module has occurred.  Please contact National Instruments technical support at ni.com/support."}, {-61498, "LabVIEW FPGA: An internal software error in the LabVIEW FPGA Module has occurred.  Please contact National Instruments technical support at ni.com/support with following information:\n\nRequired tag was not found in the resource file."}, {-61497, "LabVIEW FPGA: An internal software error in the LabVIEW FPGA Module has occurred.  Please contact National Instruments technical support at ni.com/support with following information:\n\nAn unsupported register offset was requested."}, {-61496, "LabVIEW FPGA: An internal software error in the LabVIEW FPGA Module has occurred.  Please contact National Instruments technical support at ni.com/support with following information:\n\nAn unexpected case was reached."}, {-61495, "LabVIEW FPGA: An internal software error in the LabVIEW FPGA Module has occurred.  Please contact National Instruments technical support at ni.com/support with following information:\n\nA path tag specified a value that is not a path."}, {-61494, "LabVIEW FPGA: An internal software error in the LabVIEW FPGA Module has occurred.  Please contact National Instruments technical support at ni.com/support with following information:\n\nAn IP Generator VI did not match the required interface."}, {-61493, "LabVIEW FPGA: An internal software error in the LabVIEW FPGA Module has occurred.  Please contact National Instruments technical support at ni.com/support with following information:\n\nThe specified IP Generator VI could not be found."}, {-61492, "LabVIEW FPGA: An internal software error in the LabVIEW FPGA Module has occurred.  Please contact National Instruments technical support at ni.com/support with following information:\n\nError accessing FPGA provider."}, {-61491, "LabVIEW FPGA: An internal software error in the LabVIEW FPGA Module has occurred.  Please contact National Instruments technical support at ni.com/support with following information:\n\nAn IP Generator is missing the required VI Path Tag."}, {-61490, "LabVIEW FPGA: An internal error has occurred."}, {-61489, "LabVIEW FPGA: Internal software error(s)."}, {-61488, "LabVIEW FPGA: An internal software error in the LabVIEW FPGA Module has occurred.  Please contact National Instruments technical support at ni.com/support with following information:\n\nA required XML tag was not found."}, {-61487, "LabVIEW FPGA: This channel control or indicator is on the top-level VI."}, {-61475, "LabVIEW FPGA: The XML tag \"DramAddressBitAlignment\" is missing from the target resource XML file. For more details consult LabVIEW_FPGA_PlugInManual.doc."}, {-61474, "LabVIEW FPGA: \"FFT size\" must be greater than or equal to the number of samples per input."}, {-61473, "LabVIEW FPGA: The \"imaginary data\" input array size is different from that of the \"real data\" input. The array sizes of these inputs must be the same."}, {-61472, "LabVIEW FPGA: The input array size must be 2, 4, 8, or 16."}, {-61471, "LabVIEW FPGA: You must reload the IO Module declaration file."}, {-61470, "LabVIEW FPGA: You must reload the DRAM declaration file."}, {-61469, "LabVIEW FPGA: Invalid size for Stream or Lossy Stream channel writer."}, {-61468, "LabVIEW FPGA: A channel terminal of a non-reentrant subVI is connected to multiple channels."}, {-61467, "LabVIEW FPGA: Stream or Lossy Stream writer endpoints not wired correctly."}, {-61466, "LabVIEW FPGA: LabVIEW encountered an error when trying to run the Vivado Design Suite scripts."}, {-61465, "LabVIEW FPGA: LabVIEW failed to delete a file."}, {-61464, "LabVIEW FPGA: LabVIEW failed to delete a file."}, {-61463, "LabVIEW FPGA: LabVIEW failed to export project for the Vivado Design Suite."}, {-61462, "LabVIEW FPGA: The design was unable to meet timing requirements due to a pulse width violation."}, {-61461, "LabVIEW FPGA: This version of LabVIEW does not support the requested FPGA compilation tools."}, {-61460, "LabVIEW FPGA: Control and indicator names with newline characters are only supported when the VI execution mode is set to Simulation (Simulated I/O) and the FPGA VI reference is configured for Dynamic mode."}, {-61459, "LabVIEW FPGA: The selected target requires 64-bit Xilinx tools, but the system uses a 32-bit OS."}, {-61458, "LabVIEW FPGA: Target does not support terminals configured for variable and bounded size arrays."}, {-61457, "LabVIEW FPGA: The compilation status file is missing or corrupt."}, {-61456, "LabVIEW FPGA: The FPGA design did not meet timing requirements and the source of the timing failure could not be located automatically."}, {-61455, "LabVIEW FPGA: Some of the compilation steps were not executed."}, {-61454, "LabVIEW FPGA: Some signals were not properly constrained in the design."}, {-61453, "LabVIEW FPGA: The constraints file was not used in the compilation."}, {-61452, "LabVIEW FPGA: The compilation failed due to resource overmapping."}, {-61451, "LabVIEW FPGA: The compilation failed due to timing violations."}, {-61450, "LabVIEW FPGA: The compilation failed due to a Xilinx error."}, {-61449, "LabVIEW FPGA: The FPGA VI has finished executing."}, {-61448, "LabVIEW FPGA: The simulation is not running."}, {-61447, "LabVIEW FPGA: LabVIEW cannot locate the VI."}, {-61446, "LabVIEW FPGA: The execution mode is invalid for the Desktop Execution Node."}, {-61445, "LabVIEW FPGA: The handshake is outside a single-cycle Timed Loop."}, {-61444, "LabVIEW FPGA: The Desktop Execution Node is misconfigured."}, {-61443, "LabVIEW FPGA: The simulation has exceeded the maximum simulated time."}, {-61442, "LabVIEW FPGA: The FPGA Desktop Execution Node cannot run the configured VI."}, {-61441, "LabVIEW FPGA: Another FPGA VI for this target is already executing on the development computer. Stop the other VI before running this VI."}, {-61417, "LabVIEW FPGA: The method does not support FIFOs with the \"UltraRAM\" implementation."}, {-61416, "LabVIEW FPGA: The current target does not support FIFOs with the UltraRAM implementation."}, {-61415, "LabVIEW FPGA: The method does not support FIFOs with the \"Built-In\" control logic."}, {-61414, "LabVIEW FPGA: Control or indicator data type is not supported."}, {-61413, "LabVIEW FPGA: FIFO with handshaking interface is outside a single-cycle Timed Loop."}, {-61412, "LabVIEW FPGA: Missing feedback node after Ready For Input terminal."}, {-61411, "LabVIEW FPGA: FIFO invokes methods with incompatible interfaces."}, {-61410, "LabVIEW FPGA: Target does not support the handshaking interface on this FIFO."}, {-61408, "LabVIEW FPGA: Feedback Node initialization unsupported."}, {-61406, "LabVIEW FPGA: The logic in a socketed CLIP is preventing the FPGA VI from running."}, {-61405, "LabVIEW FPGA: The operation failed because you do not have a physical target specified for this FPGA target. \n\nRight-click the FPGA target in the Project Explorer window, select Properties, and enter an FPGA target resource name in the Resource text box."}, {-61404, "LabVIEW FPGA: LabVIEW encountered a target-specific error or warning."}, {-61403, "LabVIEW FPGA: LabVIEW is unable to interact with the current target because a required file is missing or inaccessible. Check that the FPGA target-specific driver software is installed correctly."}, {-61402, "LabVIEW FPGA: LabVIEW lost communication with the device. \n\nThe resource for the target was disconnected or removed.\n\nIf the target is located remotely, the remote system might be turned off or there might be a network problem."}, {-61400, "LabVIEW FPGA: Operation failed because the type of the hardware specified in the project and/or in the VI does not match the type of the hardware that was physically accessed."}, {-61399, "LabVIEW FPGA: Execution of the FPGA VI on the development computer is not supported for the given item/node in the custom VI used for FPGA I/O."}, {-61398, "LabVIEW FPGA: FPGA VI simulation failed because either the path for the specified custom VI for FPGA I/O simulation is missing or incorrect, or the specified custom VI for FPGA I/O simulation uses an incorrect connector pane. Check the custom VI path on the Simulation page of the target settings or check that the VI matches the required interface."}, {-61397, "LabVIEW FPGA: Execution of the FPGA VI on the development computer failed because the custom VI for FPGA I/O does not conform to the calling requirements of the FPGA VI."}, {-61396, "LabVIEW FPGA: Execution of the FPGA VI on the development computer failed because the custom VI for FPGA I/O called a VI or a function that returned an error."}, {-61395, "LabVIEW FPGA: Execution of the FPGA VI on the development computer failed because the custom VI for FPGA I/O is not executable."}, {-61394, "LabVIEW FPGA: This VI is supported only when the Execution Stage is Running."}, {-61355, "LabVIEW FPGA: An internal software error has occurred. DFIR refnum not found."}, {-61354, "LabVIEW FPGA: Internal software error(s): Connected node is not constant."}, {-61353, "LabVIEW FPGA: Internal software error(s): Output terminal not supported."}, {-61352, "LabVIEW FPGA: Internal software error(s): Terminal is not connectable."}, {-61351, "LabVIEW FPGA: Internal software error(s): Terminal is unconnected."}, {-61350, "LabVIEW FPGA: Internal software error(s): Terminal Index Out of Bounds."}, {-61347, "LabVIEW FPGA: The user has reached the maximum number of simultaneous compiles for this compile cloud account."}, {-61346, "LabVIEW FPGA: The FPGA Compile Farm Server does not support the current version of the FPGA Module. Use a compatible version of the FPGA Compile Farm Server or switch to another server. Refer to the FPGA Module readme for information about FPGA Module versions supported 
